vi "Auto-name Control Panel Items.vi"(6 "Variant in":variant, 7 "Shift Pressed?":bool, 8 "error in (no error)":errorcluster, 10 "QD Combo Box Ref":refnum<vi>, 11 "QD Launch VI Ref":refnum<vi>) -> (0 "error out":errorcluster, 4 "Variant out":variant)   [LabVIEW 2017]
doc: "This plugin renames control panel items to match their class types.\n\nDefault Shortcut - [N]"
panel:
  in  "Undo Name":string="Quick Drop Keyboard Shortcut"
  # "Do not change the connector pane of this VI.\n\nSee the block diagram for directions on how to use this template."
  # "Specify the name of the Undo transaction"
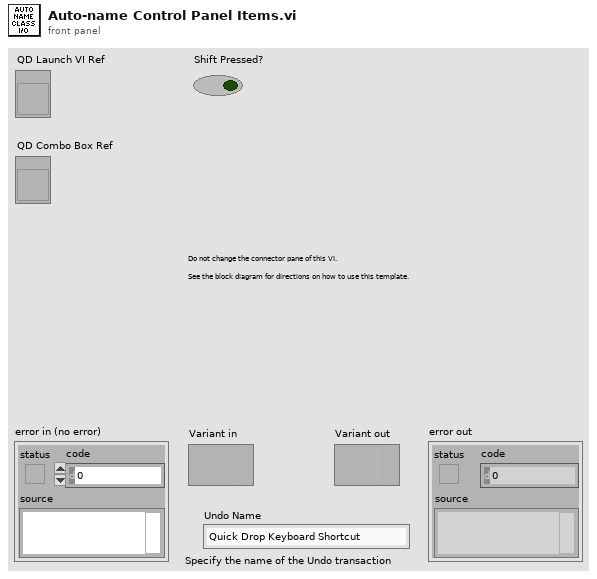
[diagram p1: front panel]
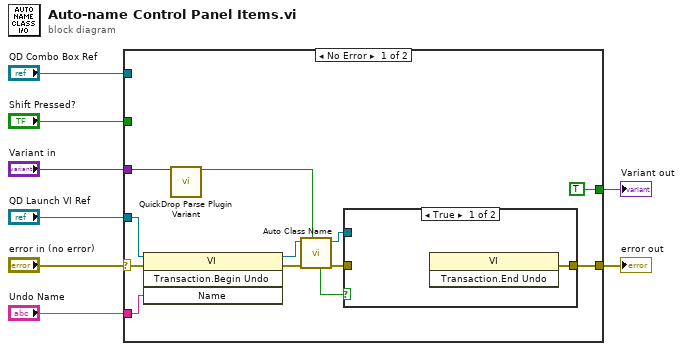
[diagram p0: block diagram]
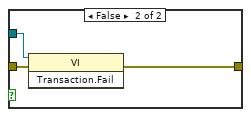
[diagram p2: hidden frame]
diagram:
  n1 = case shown="No Error" "error in (no error)" {
    selector: "error in (no error)" -> [w19 w25]
    tunnel: [w15 w25] -> w7
    tunnel: "QD Launch VI Ref" -> [w18 _]
    tunnel: "Shift Pressed?" -> [_ _]
    tunnel: "QD Combo Box Ref" -> [_ _]
    tunnel: "Variant in" -> [w20 _]
    tunnel: "Undo Name" -> [w17 _]
    tunnel: [TRUE _] -> w1
    frame No Error {
      n2 = invoke class="VI" method="Transaction.Begin Undo"(reference=w18, error in=w19, "Name"=w17) -> (reference out=w13:refnum<vi>, error out=w14:errorcluster)  [unwired: 1 in, 2 out]
      n3 = call <vilib>:"QuickDrop Parse Plugin Variant.vi"("QDKS Variant in"=w20) -> ("QD Launch VI Panel?"=w10:bool)  [unwired: 12 in, 2 out]
      n4 = call "Auto Class Name.vi"("QD Launch VI Panel?"=w10, "error in (no error)"=w14, "VI in"=w13) -> ("error out"=w12:errorcluster, "VI out"=w11:refnum<vi>, "Completed"=w9:bool)  [unwired: 6 in]
      n5 = case shown="True" w9 {
        tunnel: [w21 w24] -> w15
        tunnel: w12 -> [_ w23]
        tunnel: w11 -> [_ w22]
        frame True {
          n6 = invoke class="VI" method="Transaction.End Undo"() -> (error out=w21:errorcluster)  [unwired: 3 in, 2 out]
        }
        frame False {
          n7 = invoke class="VI" method="Transaction.Fail"(reference=w22, error in=w23) -> (error out=w24:errorcluster)  [unwired: 1 in, 2 out]
        }
      }
    }
    frame Error {
    }
  }
  "error out" <- w7
  "Variant out" <- w1
